vi "Switch Abort Q Ops on Errors.vi"(8 "error in (no error)":errorcluster, 11 "Queue":refnum<queue>) -> (0 "error out":errorcluster)   [LabVIEW 2011]
uses:
  TypeDefs/Switch Queue Cluster.ctl
  TypeDefs/Switch Test Parameters.ctl
  TypeDefs/Switch Stimulus Parameters.ctl
  TypeDefs/Switch Type.ctl
  TypeDefs/Switch Instrument Info.ctl
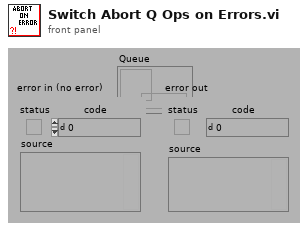
[diagram p1: front panel]
types:
  T1 = typedef "Switch Test Parameters.ctl" = cluster{"Stimulus":T2, "Switch Info":T4}
  T2 = typedef "Switch Stimulus Parameters.ctl" = cluster{"Blank Screen":bool, "SWI Position":variant, "Switch Type":T3}
  T3 = typedef "Switch Type.ctl" = enum16{"Sea-Level", "Simulator", "SI-0206-SW", "SI-0309-SW", "SI-0310-SW", "Front End"}
  T4 = typedef "Switch Instrument Info.ctl" = cluster{"sDriverId":string, "sDriverType":string, "Model":string, "Serial":string, "USB Serial":string}
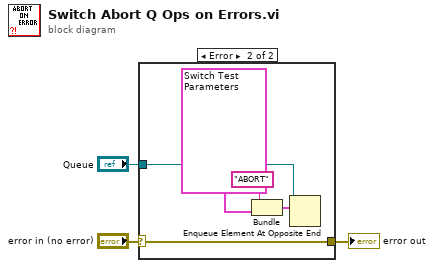
[diagram p0: block diagram]
diagram:
  n1 = case shown="Error" "error in (no error)" {
    selector: "error in (no error)" -> [w4 w8]
    tunnel: [w4 w8] -> w2
    tunnel: "Queue" -> [_ w6]
    frame No Error {
    }
    frame Error {
      n2 = Bundle("ABORT", "Test Parameters"=T1 {"Stimulus"={"Blank Screen"=FALSE, "SWI Position"=variant, "Switch Type"=enum."Sea-Level"}, "Switch Info"={"sDriverId"="", "sDriverType"="", "Model"="", "Serial"="", "USB Serial"=""}}) -> (w9:cluster{string, "Test Parameters":T1})  [unwired: 1 out]
      n3 = Enqueue Element At Opposite End(queue=w6, element=w9) -> ()  [unwired: 1 in, 4 out]
    }
  }
  "error out" <- w2
